vi "ConvertCronToSchedule.vi"(8 "error in (no error)":errorcluster, 11 "CRON expression":string) -> (0 "error out":errorcluster, 3 "chronSchedule":T1={"minutes"="*", "hours"="*", "day of month"="*", "month"="*", "day of week"="*", "year"="*"})   [LabVIEW 2017, in "CronScheduler.lvlib"]
uses:
  <vilib>/addons/InsightCM/Utilities/CronScheduler/CronScheduler.lvlib
  <vilib>/addons/InsightCM/Utilities/CronScheduler/controls/CronSchedule.ctl
  <vilib>/Utility/error.llb/whitespace.ctl
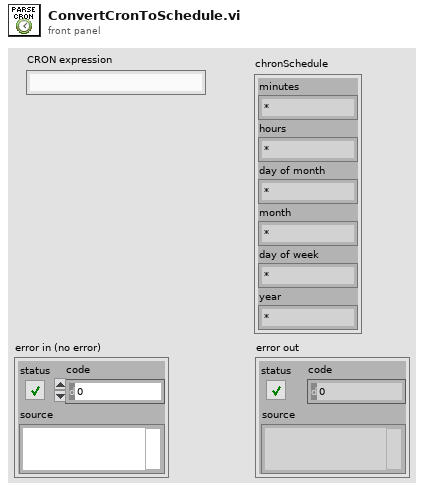
[diagram p1: front panel]
types:
  T1 = typedef "CronScheduler.lvlib/CronSchedule.ctl" = cluster{"minutes":string, "hours":string, "day of month":string, "month":string, "day of week":string, "year":string}
  T2 = typedef "whitespace.ctl" = u16
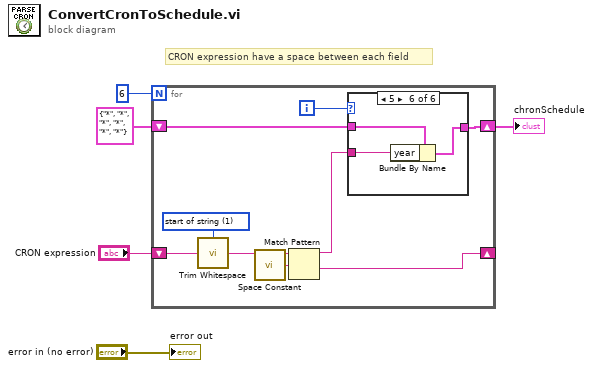
[diagram p0: block diagram]
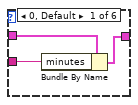
[diagram p2: hidden frame]
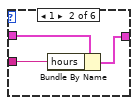
[diagram p3: hidden frame]
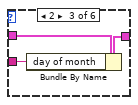
[diagram p4: hidden frame]
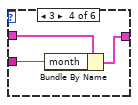
[diagram p5: hidden frame]
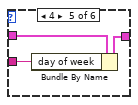
[diagram p6: hidden frame]
diagram:
  # "CRON expression have a space between each field"
  n1 = for {
    N: 6 -> [_]
    shift-right: [w10] -> _
    shift-left: "CRON expression" -> [w14]
    shift-right: [w7] -> w4
    shift-left: T1 {"minutes"="*", "hours"="*", "day of month"="*", "month"="*", "day of week"="*", "year"="*"} ("chronSchedule") -> [w8]
    i -> [w9]
    w13 = T2 1 items=["both", "start of string", "end of string"] ("location (both)")
    n2 = call <vilib>:"Trim Whitespace.vi"("string"=w14, "location (both)"=w13) -> ("trimmed string"=w12:string)
    n3 = call <vilib>:"Space Constant.vi"() -> ("String"=w11:string)
    n4 = Match Pattern(string=w12, regular expression=w11) -> (before substring=w6:string, after substring=w10:string)  [unwired: 1 in, 2 out]
    n5 = case shown="5" w9 {
      tunnel: w8 -> [w17 w20 w23 w26 w29 w32]
      tunnel: [w16 w19 w22 w25 w28 w31] -> w7
      tunnel: w6 -> [w15 w18 w21 w24 w27 w30]
      frame 0, Default {
        n6 = Bundle By Name(cluster=w17, "minutes"=w15) -> (w16:T1)
      }
      frame 1 {
        n7 = Bundle By Name(cluster=w20, "hours"=w18) -> (w19:T1)
      }
      frame 2 {
        n8 = Bundle By Name(cluster=w23, "day of month"=w21) -> (w22:T1)
      }
      frame 3 {
        n9 = Bundle By Name(cluster=w26, "month"=w24) -> (w25:T1)
      }
      frame 4 {
        n10 = Bundle By Name(cluster=w29, "day of week"=w27) -> (w28:T1)
      }
      frame 5 {
        n11 = Bundle By Name(cluster=w32, "year"=w30) -> (w31:T1)
      }
    }
  }
  "chronSchedule" <- w4
  "error out" <- "error in (no error)"
